vi "Display New Configuration SubPanel.vi"(8 "error in (no error)":errorcluster, 10 "ListBox Selection":i32, 11 "Configuration in":refnum<class "Configuration.lvclass">) -> (0 "error out":errorcluster, 3 "Configuration out":refnum<class "Configuration.lvclass">)   [LabVIEW 2017, in "Configuration.lvlib" / "Configuration.lvclass"]
uses:
  Configuration.lvclass
  Configuration.lvclass/Configuration.ctl
panel:
  out "error out 2":errorcluster
  out "VI Name":string
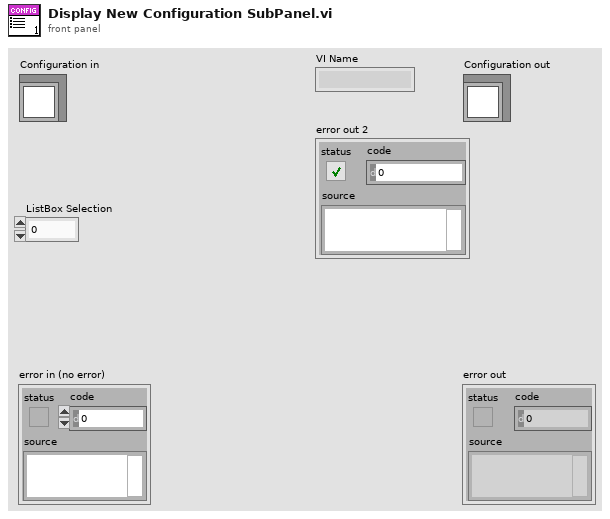
[diagram p1: front panel]
types:
  T1 = enum8{"Enabled", "Disabled", "Disabled and Grayed Out"}
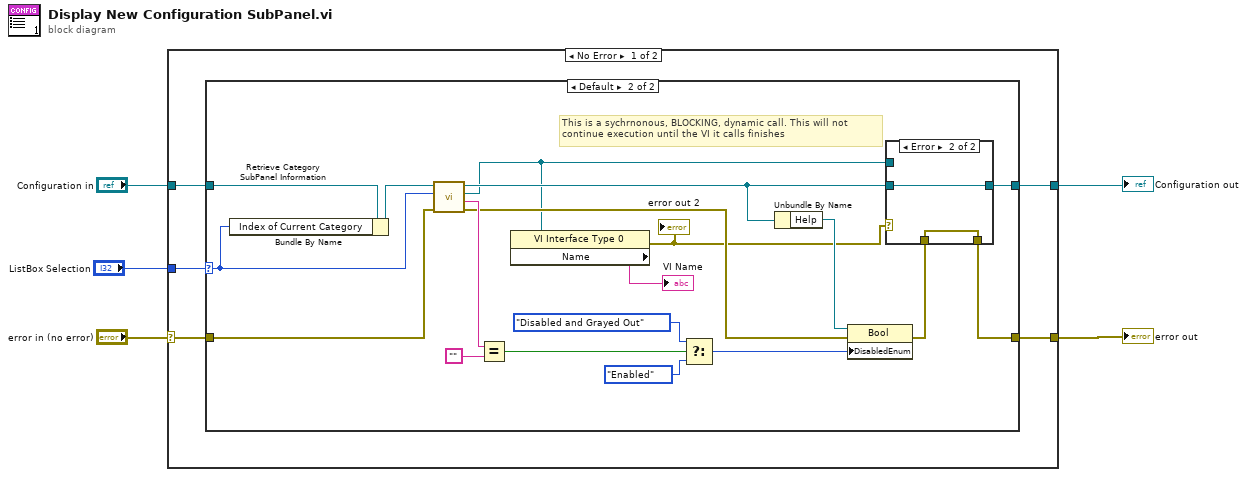
[diagram p0: block diagram]
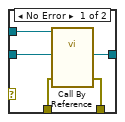
[diagram p3: hidden frame]
diagram:
  n1 = case shown="No Error" "error in (no error)" {
    selector: "error in (no error)" -> [w9 w40]
    tunnel: [w8 w40] -> w4
    tunnel: [w10 w39] -> w2
    tunnel: "Configuration in" -> [w7 w39]
    tunnel: "ListBox Selection" -> [w6 _]
    frame No Error {
      n2 = case shown="Default" w6 {
        selector: w6 -> [_ w16]
        tunnel: [w12 w31] -> w10
        tunnel: w9 -> [w11 w30]
        tunnel: [w11 w29] -> w8
        tunnel: w7 -> [w12 w28]
        frame -1 {
        }
        frame Default {
          # "This is a sychrnonous, BLOCKING, dynamic call. This will not\ncontinue execution until the VI it calls finishes"
          n3 = Bundle By Name(cluster=w28, "Index of Current Category"=w16) -> (w27:refnum<class "Configuration.lvclass">)
          n4 = call "Retrieve Category SubPanel Information.vi"("error in (no error)"=w30, "ListBox Selection"=w16, "Configuration in"=w27) -> ("error out"=w17:errorcluster, "Help Text"=w24:string, "VI Refnum"=w15:refnum<vi>, "Configuration Out"=w26:refnum<class "Configuration.lvclass">)  [unwired: 5 in]
          n5 = Equal?(x=w24, y="") -> (x = y?=w21:bool)
          n6 = property class="VI Interface Type 0"(reference=w15) -> (error out=w13:errorcluster, "Name"=→"VI Name":string)  [unwired: 1 in, 1 out]
          "error out 2" <- w13
          n7 = Select(t=T1."Disabled and Grayed Out" ("Disabled"), s=w21, f=T1."Enabled" ("Disabled")) -> (s? t:f=w20:T1)
          n8 = Unbundle By Name(w26) -> ("Help"=w23:refnum<vi>)
          n9 = property class="Bool"(reference=w23, error in=w17, "DisabledEnum"=w20) -> (error out=w22:errorcluster)  [unwired: 1 out]
          n10 = case shown="Error" w13 {
            tunnel: [w36 w38] -> w31
            tunnel: [w35 w37] -> w29
            tunnel: w26 -> [w34 w38]
            tunnel: w22 -> [w33 w37]
            tunnel: w15 -> [w32 _]
            frame No Error {
              n11 = call-by-ref "?"(reference=w32, "error in (no error)"=w33, "Configuration in"=w34) -> ("error out"=w35:errorcluster, "Configuration out"=w36:refnum<class "Configuration.lvclass">)  [unwired: 9 in, 2 out]
            }
            frame Error {
            }
          }
        }
      }
    }
    frame Error {
    }
  }
  "error out" <- w4
  "Configuration out" <- w2
